vi "I16_to_BSON_bytes.vi"(11 "value":i16) -> (3 "BSONbytes":u8[](array[numeric]))   [LabVIEW 2015, in "BSON_convertors_Library.lvlib"]
doc: "Created by Artem Shevelev\nLabVIEW Portal profile: http://www.labviewportal.org/memberlist.php?mode=viewprofile&u=2340\ne-mail: artem.sh@gmail.com\nshevelev.pro"
uses:
  BSON_convertors_Library.lvlib
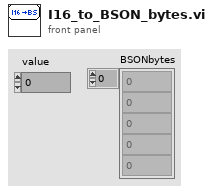
[diagram p1: front panel]
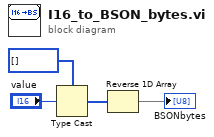
[diagram p0: block diagram]
diagram:
  n1 = Type Cast(type=u8[] [] ("*(type *) &x"), x="value") -> (*(type *) &x=w3:u8[])
  n2 = Reverse 1D Array(array=w3) -> (reversed array=→"BSONbytes":u8[])
